vi "OpenG Delete Elements from Array 2D Template.vi"(8 "delete (rows or columns)":enum16{"rows", "columns"}(ring), 9 "indices":i32[](array[numeric]), 11 "array":dbl[][](array[numeric]) format="%.2f") -> (1 "deleted elements":dbl[][](array[numeric]) format="%.2f", 3 "array w/ subset deleted":dbl[][](array[numeric]) format="%.2f")   [LabVIEW 2012]
doc: "This polymorphic VI deletes elements from a 1D or 2D <B>array</B> at the corresponding <B>indices</B>, returning <B>array w/ subset deleted</B> and <B>deleted elements</B>. For 2D arrays, wire the <B>delete (rows or columns)</B> input to specify whether to delete rows or columns."
panel:
  # "[OpenG VI Tags] ***Do Not Remove*** \nSVN Revision = 990\nSVN Revision Date = 2009-07-18 07:14:13 -0700 (Sat, 18 Jul 2009)\nPackage = oglib_array-3.0.0-1\nDepends ="
  # "Delete Elements from Array.vi\n\nThis polymorphic VI deletes elements from a 1D or 2D array at the corresponding indices\n\nPlease visit http://www.OpenG.org to learn about the\nOpen Source LabVIEW software movement.\n\nNOTICE -- YOU MUST LEAVE THIS NOTICE IN PLACE.  PER THE TERMS OF THE LICENSE BELOW, YOU MAY SUBLICENSE THIS SOFTWARE \nIN ANY WAY THAT DOES NOT CONFLICT WITH THIS LICENSE.\n\n### BSD License (http://www.opensource.org/licenses/bsd-license.php) Begin ###\n \nCopyright (c) 2007, JKI <info@jameskring.com> (Author: Jim Kring <jim.kring@jameskring.com>)\n\nAll rights reserved.\n\nRedistribution and use in source and binary forms, with or without modification, are permitted provided that the following conditions are met:\n\n    * Redistributions of source code must retain the above copyright notice, this list of conditions and the following disclaimer.\n    * Redistributions in binary form must reproduce the above copyright notice, this list of conditions and the following disclaimer in the \n       documentation and/or other materials provided with the distribution.\n    * Neither the name of SciWare, James Kring, Inc., nor the names of its contributors may be used to endorse or promote products derived \n       from this software without specific prior written permission.\n\nTHIS SOFTWARE IS PROVIDED BY THE COPYRIGHT HOLDERS AND CONTRIBUTORS \"AS IS\" AND ANY EXPRESS OR IMPLIED WARRANTIES, \nINCLUDING, BUT NOT LIMITED TO, THE IMPLIED WARRANTIES OF MERCHANTABILITY AND FITNESS FOR A PARTICULAR PURPOSE ARE \nDISCLAIMED. IN NO EVENT SHALL THE COPYRIGHT OWNER OR CONTRIBUTORS BE LIABLE FOR ANY DIRECT, INDIRECT, INCIDENTAL,\n SPECIAL, EXEMPLARY, OR CONSEQUENTIAL DAMAGES (INCLUDING, BUT NOT LIMITED TO, PROCUREMENT OF SUBSTITUTE GOODS OR \nSERVICES; LOSS OF USE, DATA, OR PROFITS; OR BUSINESS INTERRUPTION) HOWEVER CAUSED AND ON ANY THEORY OF LIABILITY, \nWHETHER IN CONTRACT, STRICT LIABILITY, OR TORT (INCLUDING NEGLIGENCE OR OTHERWISE) ARISING IN ANY WAY OUT OF THE USE \nOF THIS SOFTWARE, EVEN IF ADVISED OF THE POSSIBILITY OF SUCH DAMAGE.\n\n### BSD License End ###"
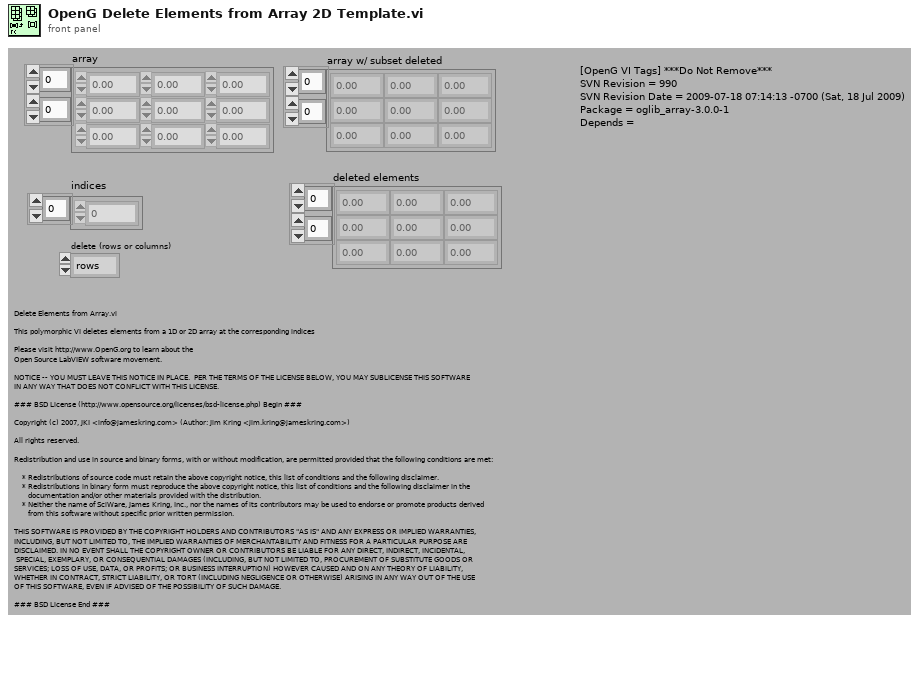
[diagram p1: front panel]
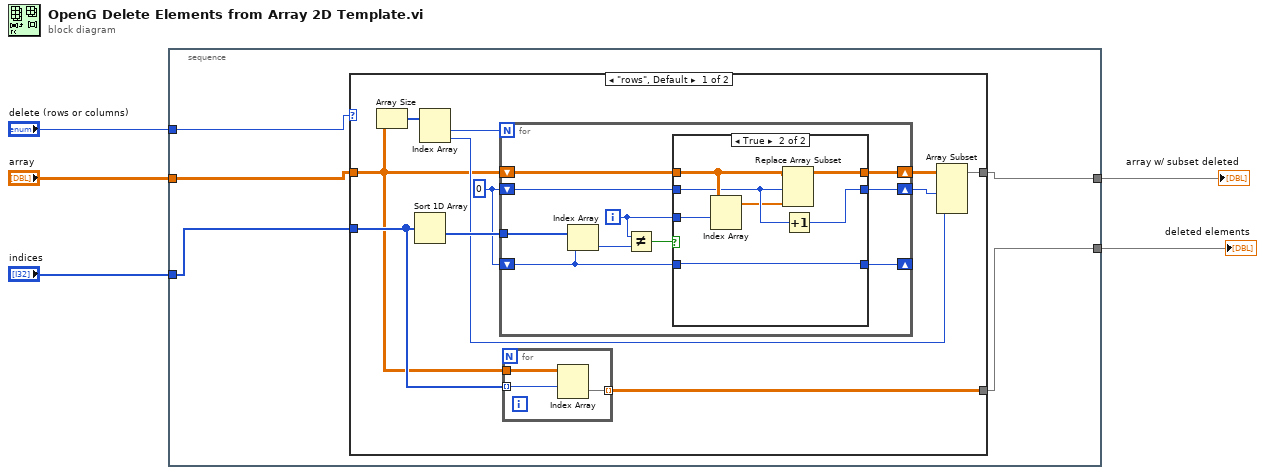
[diagram p0: block diagram]
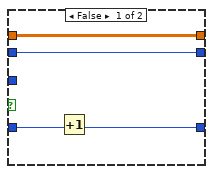
[diagram p2: hidden frame]
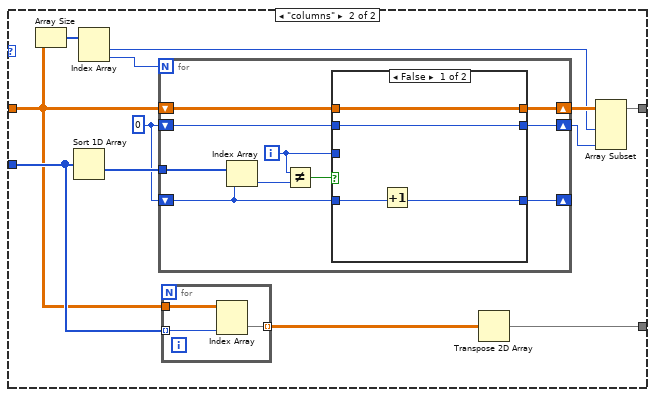
[diagram p3: hidden frame]
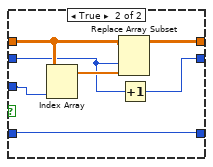
[diagram p4: hidden frame]
diagram:
  n1 = stacked-sequence {
    tunnel: [w7] -> w5
    tunnel: "delete (rows or columns)" -> [w10]
    tunnel: "indices" -> [w8]
    tunnel: "array" -> [w9]
    tunnel: [w6] -> w1
    frame #0 {
      n2 = case shown="\"rows\", Default" w10 {
        tunnel: w8 -> [w20 w57]
        tunnel: [w21 w47] -> w6
        tunnel: w9 -> [w13 w53]
        tunnel: [w11 w48] -> w7
        frame "rows", Default {
          w12 = 0
          n3 = Array Size(array=w13) -> (size(s)=w19:i32[])
          n4 = Sort 1D Array(array=w20) -> (sorted array=w18:i32[])
          n5 = Index Array(array=w19) -> (element #1=w15:i32, element #2=w14:i32)  [unwired: 2 in]
          n6 = for {
            N: w15 -> [_]
            shift-right: [w24] -> w17
            shift-left: w13 -> [w28]
            shift-right: [w25] -> w16
            shift-left: w12 -> [w26]
            shift-right: [w23] -> _
            shift-left: w12 -> [w22]
            tunnel: w18 -> [w31]
            i -> [w27]
            n7 = Index Array(array=w31, index=w22) -> (element=w30:i32)
            n8 = Not Equal?(x=w27, y=w30) -> (x != y?=w29:bool)
            n9 = case shown="True" w29 {
              tunnel: w28 -> [w34 w41]
              tunnel: w27 -> [_ w42]
              tunnel: w26 -> [w33 w40]
              tunnel: [w33 w39] -> w25
              tunnel: [w34 w38] -> w24
              tunnel: w22 -> [w35 w36]
              tunnel: [w32 w36] -> w23
              frame False {
                n10 = Increment(x=w35) -> (x+1=w32:i32)
              }
              frame True {
                n11 = Index Array(array=w41, index (row)=w42) -> (element=w37:dbl[])  [unwired: 1 in]
                n12 = Replace Array Subset(array=w41, new element=w37, index (row)=w40) -> (w38:dbl[][])  [unwired: 1 in]
                n13 = Increment(x=w40) -> (x+1=w39:i32)
              }
            }
          }
          n14 = for {
            tunnel: w20 -> [w44] mode=indexing
            tunnel: w13 -> [w45]
            tunnel: [w43] -> w21 mode=indexing
            n15 = Index Array(array=w45, index (row)=w44) -> (element=w43:dbl[])  [unwired: 1 in]
          }
          n16 = Array Subset(array=w17, length (row)=w16, length (col)=w14) -> (w11:dbl[][])  [unwired: 2 in]
        }
        frame "columns" {
          w52 = 0
          n17 = Array Size(array=w53) -> (size(s)=w56:i32[])
          n18 = Sort 1D Array(array=w57) -> (sorted array=w55:i32[])
          n19 = Index Array(array=w56) -> (element #1=w50:i32, element #2=w51:i32)  [unwired: 2 in]
          n20 = for {
            N: w51 -> [_]
            shift-right: [w60] -> w54
            shift-left: w53 -> [w64]
            shift-right: [w61] -> w49
            shift-left: w52 -> [w62]
            shift-right: [w59] -> _
            shift-left: w52 -> [w58]
            tunnel: w55 -> [w67]
            i -> [w63]
            n21 = Index Array(array=w67, index=w58) -> (element=w66:i32)
            n22 = Not Equal?(x=w63, y=w66) -> (x != y?=w65:bool)
            n23 = case shown="False" w65 {
              tunnel: w64 -> [w70 w78]
              tunnel: w63 -> [_ w73]
              tunnel: w62 -> [w69 w72]
              tunnel: [w69 w77] -> w61
              tunnel: [w70 w76] -> w60
              tunnel: w58 -> [w71 w74]
              tunnel: [w68 w74] -> w59
              frame False {
                n24 = Increment(x=w71) -> (x+1=w68:i32)
              }
              frame True {
                n25 = Index Array(array=w78, index (col)=w73) -> (element=w75:dbl[])  [unwired: 1 in]
                n26 = Replace Array Subset(array=w78, new element=w75, index (col)=w72) -> (w76:dbl[][])  [unwired: 1 in]
                n27 = Increment(x=w72) -> (x+1=w77:i32)
              }
            }
          }
          n28 = for {
            tunnel: w57 -> [w79] mode=indexing
            tunnel: w53 -> [w81]
            tunnel: [w80] -> w46 mode=indexing
            n29 = Index Array(array=w81, index (col)=w79) -> (element=w80:dbl[])  [unwired: 1 in]
          }
          n30 = Transpose 2D Array(2D array=w46) -> (transposed array=w47:dbl[][])
          n31 = Array Subset(array=w54, length (row)=w50, length (col)=w49) -> (w48:dbl[][])  [unwired: 2 in]
        }
      }
    }
  }
  "array w/ subset deleted" <- w5
  "deleted elements" <- w1
